vi "Select Active Refs (SubVI).vi"(0 "Label Text":string, 7 "(A) Refs":T1, 9 "(B) Refs":T1, 11 "(C) Refs":T1) -> (8 "Active Refs":T1)   [LabVIEW 2010]
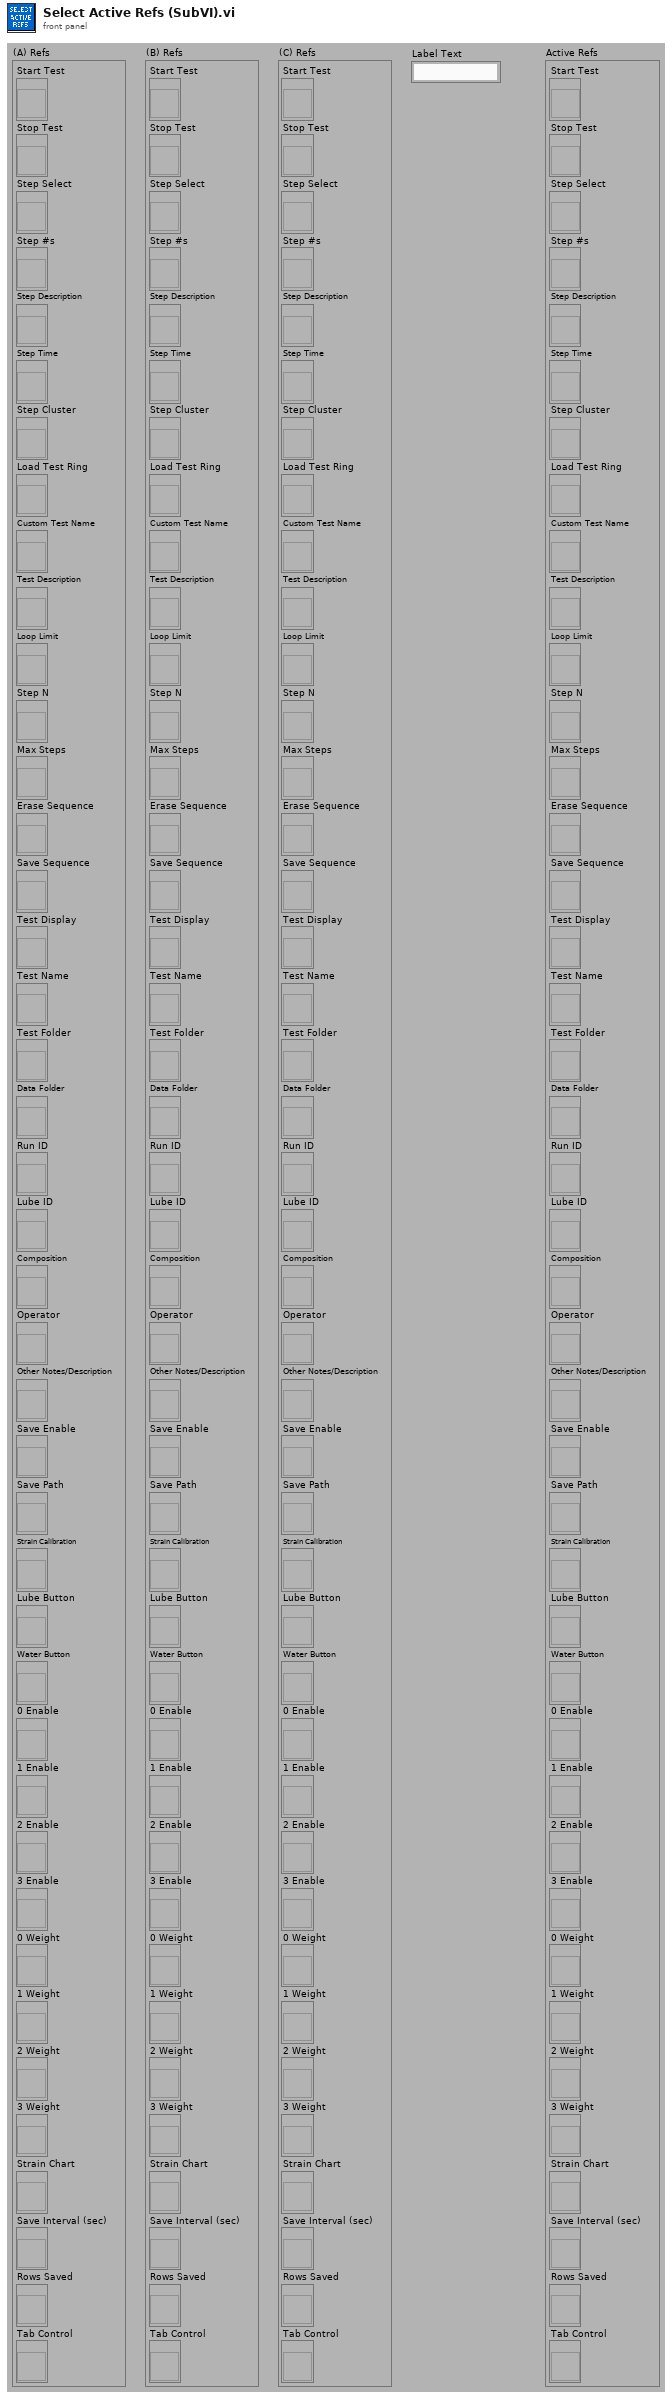
[diagram p1: front panel]
types:
  T1 = cluster{"Start Test":refnum<vi>, "Stop Test":refnum<vi>, "Step Select":refnum<vi>, "Step #s":refnum<vi>, "Step Description":refnum<vi>, "Step Time":refnum<vi>, "Step Cluster":refnum<vi>, "Load Test Ring":refnum<vi>, "Custom Test Name":refnum<vi>, "Test Description":refnum<vi>, "Loop Limit":refnum<vi>, "Step N":refnum<vi>, "Max Steps":refnum<vi>, "Erase Sequence":refnum<vi>, "Save Sequence":refnum<vi>, "Test Display":refnum<vi>, "Test Name":refnum<vi>, "Test Folder":refnum<vi>, "Data Folder":refnum<vi>, "Run ID":refnum<vi>, "Lube ID":refnum<vi>, "Composition":refnum<vi>, "Operator":refnum<vi>, "Other Notes/Description":refnum<vi>, "Save Enable":refnum<vi>, "Save Path":refnum<vi>, "Strain Calibration":refnum<vi>, "Lube Button":refnum<vi>, "Water Button":refnum<vi>, "0 Enable":refnum<vi>, "1 Enable":refnum<vi>, "2 Enable":refnum<vi>, "3 Enable":refnum<vi>, "0 Weight":refnum<vi>, "1 Weight":refnum<vi>, "2 Weight":refnum<vi>, "3 Weight":refnum<vi>, "Strain Chart":refnum<vi>, "Save Interval (sec)":refnum<vi>, "Rows Saved":refnum<vi>, "Tab Control":refnum<vi>}
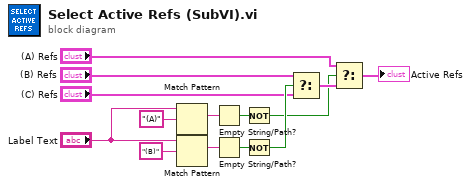
[diagram p0: block diagram]
diagram:
  n1 = Match Pattern(string="Label Text", regular expression="(A)") -> (match substring=w2:string)  [unwired: 1 in, 3 out]
  n2 = Match Pattern(string="Label Text", regular expression="(B)") -> (match substring=w5:string)  [unwired: 1 in, 3 out]
  n3 = Empty String/Path?(string/path=w2) -> (empty?=w3:bool)
  n4 = Empty String/Path?(string/path=w5) -> (empty?=w6:bool)
  n5 = Not(x=w3) -> (.not. x?=w8:bool)
  n6 = Not(x=w6) -> (.not. x?=w12:bool)
  n7 = Select(t="(B) Refs", s=w12, f="(C) Refs") -> (s? t:f=w9:T1)
  n8 = Select(t="(A) Refs", s=w8, f=w9) -> (s? t:f=→"Active Refs":T1)
